vi "GUItoPLCfloat.vi"() -> ()   [LabVIEW 2023]
panel:
  out "DB Output Array":u32[](array[numeric])
  out "Array":bool[](array[boolean])
  in  "Real Input Array":dbl[](array[numeric])
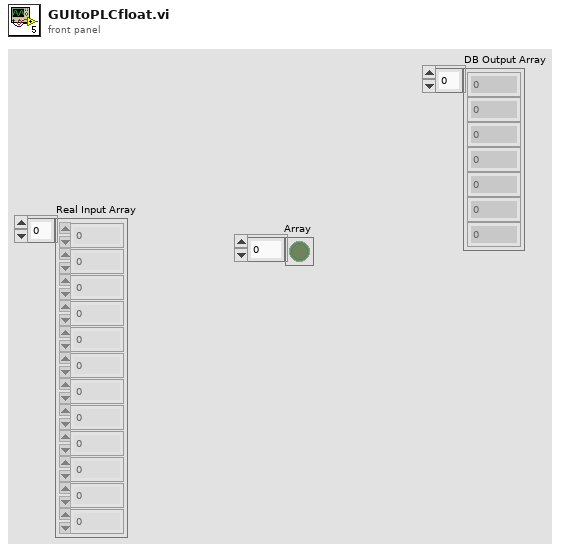
[diagram p1: front panel]
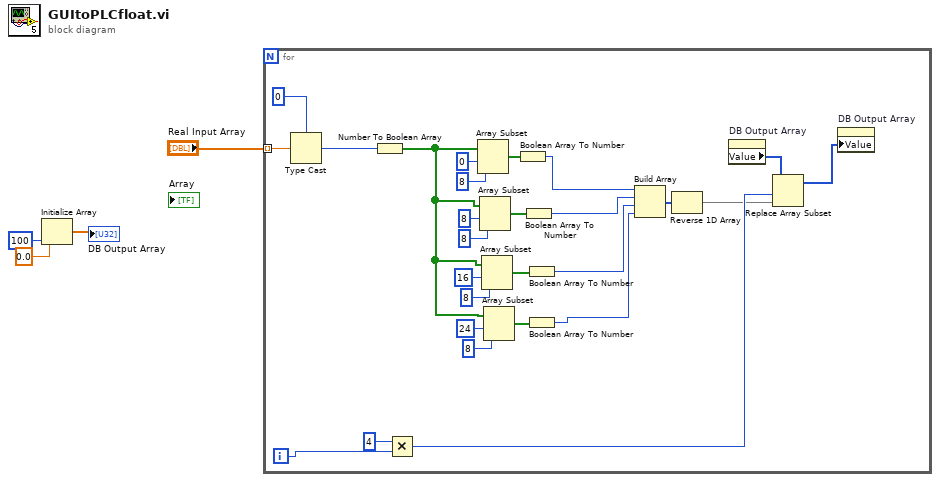
[diagram p0: block diagram]
diagram:
  n1 = Initialize Array(0.0 ("element"), 100 ("dimension size")) -> (→"DB Output Array":dbl[])
  n2 = for {
    tunnel: "Real Input Array" -> [w31] mode=indexing
    i -> [w9]
    n3 = Type Cast(type=0, x=w31) -> (*(type *) &x=w29:i32)
    n4 = Number To Boolean Array(number=w29) -> (Boolean array=w20:bool[])
    n5 = Multiply(x=4, y=w9) -> (x*y=w8:i32)
    n6 = Array Subset(array=w20, index=0, length=8) -> (w19:bool[])
    n7 = Array Subset(array=w20, index=8, length=8) -> (w17:bool[])
    n8 = Array Subset(array=w20, index=16, length=8) -> (w16:bool[])
    n9 = Array Subset(array=w20, index=24, length=8) -> (w18:bool[])
    n10 = Boolean Array To Number(Boolean array=w19) -> (number=w15:u32)
    n11 = Boolean Array To Number(Boolean array=w17) -> (number=w14:u32)
    n12 = Boolean Array To Number(Boolean array=w16) -> (number=w13:u32)
    n13 = Boolean Array To Number(Boolean array=w18) -> (number=w12:u32)
    n14 = Build Array(w15, w14, w13, w12) -> (w6:u32[])
    n15 = Reverse 1D Array(array=w6) -> (reversed array=w5:u32[])
    n16 = property on="DB Output Array" class="Arr (strict)"() -> ("Value"=w11:u32[])  [unwired: 2 in, 2 out]
    n17 = Replace Array Subset(array=w11, new element=w5, index=w8) -> (w10:u32[])
    n18 = property on="DB Output Array" class="Arr (strict)"("Value"=w10) -> ()  [unwired: 2 in, 2 out]
  }
